vi "ToPane.vi"(8 "error in":errorcluster, 11 "Generic":refnum<class "Generic.lvclass">) -> (0 "error out":errorcluster, 3 "Pane out":refnum<class "Pane.lvclass">)   [LabVIEW 2014, in "Raspberry Pi Compatible Compiler for LabVIEW.lvlib" / "Pane.lvclass"]
uses:
  Pane.lvclass
  Generic/Generic.lvclass
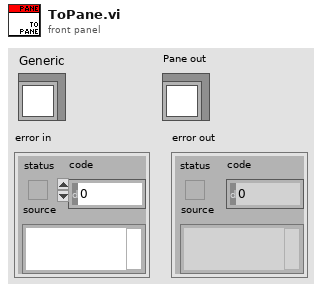
[diagram p1: front panel]
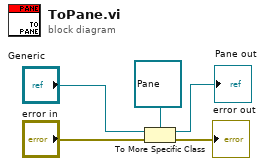
[diagram p0: block diagram]
diagram:
  n1 = To More Specific Class(target class=refnum<class "Pane.lvclass"> refnum ("Pane in"), reference="Generic", error in="error in") -> (specific class reference=→"Pane out":refnum<class "Pane.lvclass">, error out=→"error out":errorcluster)
